vi "readFromXML.vi"(8 "error in (no error)":errorcluster, 10 "XML in":string, 11 "CommandsForAllAxes in":refnum<class "CommandsForAllAxes.lvclass">) -> (0 "error out":errorcluster, 3 "CommandsForAllAxes out":refnum<class "CommandsForAllAxes.lvclass">)   [LabVIEW 2014, in "TCSDataDefinitions.lvlib" / "TCSMountControlCommand.lvlib" / "CommandsForAllAxes.lvlib" / "CommandsForAllAxes.lvclass"]
uses:
  CommandsForAllAxes.lvclass
  TCSMCCCommand/TCSMCCCommand.lvclass
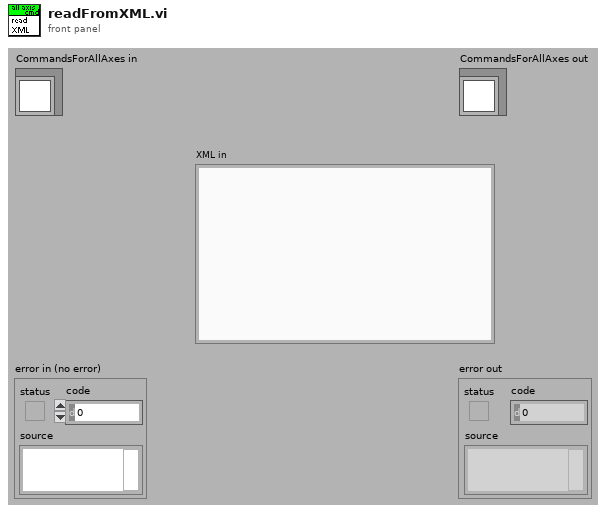
[diagram p1: front panel]
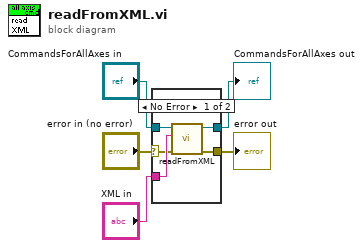
[diagram p0: block diagram]
diagram:
  n1 = case shown="No Error" "error in (no error)" {
    selector: "error in (no error)" -> [w8 w12]
    tunnel: [w6 w12] -> w4
    tunnel: [w7 w11] -> w2
    tunnel: "CommandsForAllAxes in" -> [w10 w11]
    tunnel: "XML in" -> [w9 _]
    frame No Error {
      n2 = call-parent "readFromXML.vi"("error in (no error)"=w8, "XML in"=w9, "TCSMCCCommand in"=w10) -> ("error out"=w6:errorcluster, "TCSMCCCommand out"=w7:refnum<class "CommandsForAllAxes.lvclass">)  [unwired: 7 out]
    }
    frame Error {
    }
  }
  "error out" <- w4
  "CommandsForAllAxes out" <- w2
